vi "get_ID.vi"(4 "temps d'observation (ms)":u32=300, 6 "Log?":bool, 8 "errin":errorcluster, 10 "ChannelIn":T2, 11 "Identifier":u32 format="%x") -> (0 "errout":errorcluster, 1 "trouvé":bool, 2 "TimeStampOut":T1, 3 "Messout":T3)   [LabVIEW 2020]
uses:
  C/Program Files (x86)/National Instruments/LabVIEW 2020/user.lib/PCAN Basic/Controls/Channel.ctl
  FGV.ctl
  PCANBasic.dll
  C/Program Files (x86)/National Instruments/LabVIEW 2020/user.lib/PCAN Basic/PCANBasic.lvlib
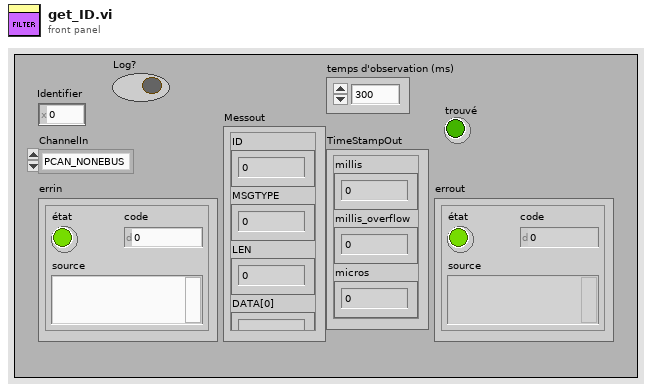
[diagram p1: front panel]
types:
  T1 = cluster{"millis":u32, "millis_overflow":u16, "micros":u16}
  T2 = typedef "PCANBasic.lvlib/Channel.ctl" = enum16{"PCAN_NONEBUS", "not used1", "not used2", "not used3", "not used4", "not used5", "not used6", "not used7", "not used8", "not used9", "not used10", "not used11", "not used12", "not used13", "not used14", "not used15", "not used16", "not used17", "not used18", "not used19", "not used20", "not used21", "not used22", "not used23", "not used24", "not used25", "not used26", "not used27", "not used28", "not used29", "not used30", "not used31", "not used32", "PCAN_ISABUS1", "PCAN_ISABUS2", "PCAN_ISABUS3", "PCAN_ISABUS4", "PCAN_ISABUS5", "PCAN_ISABUS6", "PCAN_ISABUS7", "PCAN_ISABUS8", "not used41", "not used42", "not used43", "not used44", "not used45", "not used46", "not used47", "not used48", "PCAN_DNGBUS1", "not used50", "not used51", "not used52", "not used53", "not used54", "not used55", "not used56", "not used57", "not used58", "not used59", "not used60", "not used61", "not used62", "not used63", "not used64", "PCAN_PCIBUS1", "PCAN_PCIBUS2", "PCAN_PCIBUS3", "PCAN_PCIBUS4", "PCAN_PCIBUS5", "PCAN_PCIBUS6", "PCAN_PCIBUS7", "PCAN_PCIBUS8", "not used73", "not used74", "not used75", "not used76", "not used77", "not used78", "not used79", "not used80", "PCAN_USBBUS1", "PCAN_USBBUS2", "PCAN_USBBUS3", "PCAN_USBBUS4", "PCAN_USBBUS5", "PCAN_USBBUS6", "PCAN_USBBUS7", "PCAN_USBBUS8", "Not used89", "Not used90", "Not used91", "Not used92", "Not used93", "Not used94", "Not used95", "Not used96", "PCAN_PCCBUS1", "PCAN_PCCBUS2"}
  T3 = cluster{"ID":u32, "MSGTYPE":u8, "LEN":u8, "DATA[0]":u8, "DATA[1]":u8, "DATA[2]":u8, "DATA[3]":u8, "DATA[4]":u8, "DATA[5]":u8, "DATA[6]":u8, "DATA[7]":u8}
  T4 = typedef "FGV.ctl" = enum16{"GET", "SET", "RAZ"}
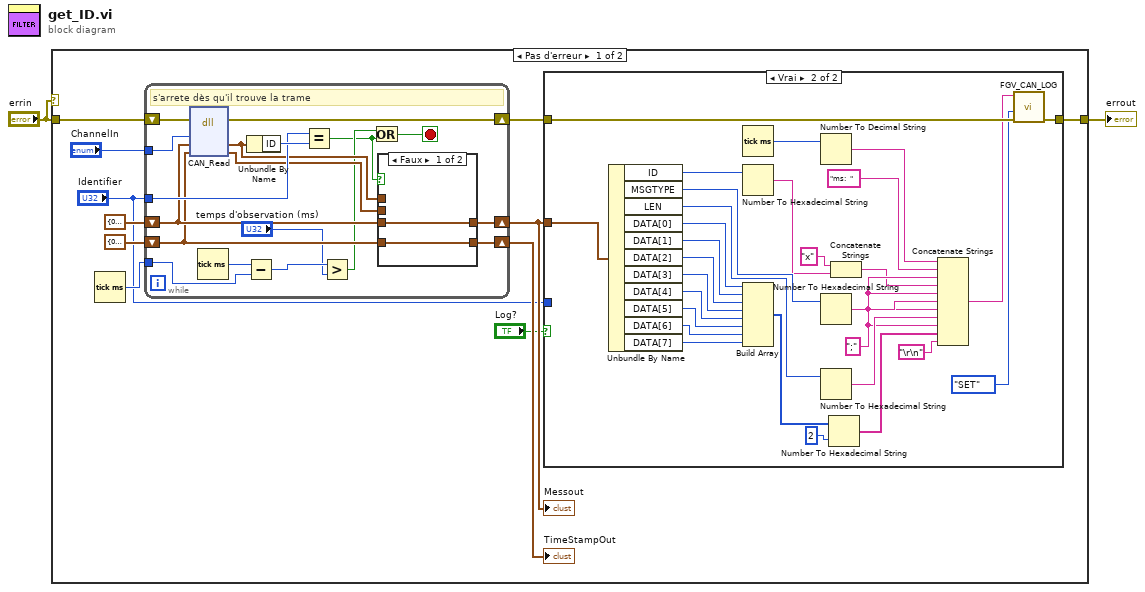
[diagram p0: block diagram]
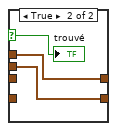
[diagram p3: hidden frame]
diagram:
  n1 = case shown="Pas d'erreur" "errin" {
    tunnel: "errin" -> [w13 w67]
    tunnel: [w6 w67] -> w2
    frame No Error {
      n2 = Tick Count (ms)() -> (millisecond timer value=w8:u32)
      n3 = while {
        tunnel: "ChannelIn" -> [w61]
        shift-right: [w59] -> w7
        shift-left: w13 -> [w60]
        tunnel: "Identifier" -> [w57]
        shift-right: [w56] -> w5
        shift-left: T3 {"ID"=0, "MSGTYPE"=0, "LEN"=0, "DATA[0]"=0, "DATA[1]"=0, "DATA[2]"=0, "DATA[3]"=0, "DATA[4]"=0, "DATA[5]"=0, "DATA[6]"=0, "DATA[7]"=0} ("MessageBuffer out") -> [w54]
        shift-right: [w55] -> w9
        shift-left: T1 {"millis"=0, "millis_overflow"=0, "micros"=0} ("TimestampBuffer out 2") -> [w53]
        tunnel: w8 -> [w50]
        stop <- w44 stop-if-true
        # "s'arrete dès qu'il trouve la trame"
        n4 = dll-call lib="PCANBasic.*" fn="CAN_Read"(error in=w60, "Channel"=w61, "MessageBuffer out"=w54, "TimestampBuffer out 2"=w53) -> (error out=w59:errorcluster, "MessageBuffer out"=w52:T3, "TimestampBuffer out 2"=w47:T1)  [unwired: 4 in, 1 out]
        n5 = Tick Count (ms)() -> (millisecond timer value=w51:u32)
        n6 = Subtract(x=w51, y=w50) -> (x-y=w49:u32)
        n7 = Unbundle By Name(w52) -> ("ID"=w58:u32)
        n8 = Equal?(x=w57, y=w58) -> (x = y?=w45:bool)
        n9 = Greater?(x=w49, y="temps d'observation (ms)") -> (0:w46:bool)
        n10 = Or(x=w46, y=w45) -> (x .or. y?=w44:bool)
        n11 = case shown="Faux" w45 {
          selector: w45 -> [_ w64]
          tunnel: w54 -> [w63 _]
          tunnel: [w63 w66] -> w56
          tunnel: [w62 w65] -> w55
          tunnel: w53 -> [w62 _]
          tunnel: w52 -> [_ w66]
          tunnel: w47 -> [_ w65]
          frame False {
          }
          frame True {
            "trouvé" <- w64
          }
        }
      }
      "Messout" <- w5
      "TimeStampOut" <- w9
      n12 = case shown="Vrai" "Log?" {
        tunnel: w7 -> [w14 w43]
        tunnel: [w14 w42] -> w6
        tunnel: w5 -> [_ w41]
        tunnel: "Identifier" -> [_ _]
        frame False {
        }
        frame True {
          w21 = ";" ("chaîne")
          n13 = Unbundle By Name(w41) -> ("ID"=w40:u32, "MSGTYPE"=w38:u8, "LEN"=w37:u8, "DATA[0]"=w34:u8, "DATA[1]"=w33:u8, "DATA[2]"=w32:u8, "DATA[3]"=w31:u8, "DATA[4]"=w30:u8, "DATA[5]"=w27:u8, "DATA[6]"=w28:u8, "DATA[7]"=w29:u8)
          n14 = Tick Count (ms)() -> (millisecond timer value=w39:u32)
          n15 = Number To Hexadecimal String(2:w40) -> (0:w16:string)  [unwired: 1 in]
          n16 = Build Array(w34, w33, w32, w31, w30, w27, w28, w29) -> (w25:u8[])
          n17 = Number To Decimal String(number=w39) -> (decimal integer string=w20:string)  [unwired: 1 in]
          n18 = Number To Hexadecimal String(2:w38) -> (0:w36:string)  [unwired: 1 in]
          n19 = Number To Hexadecimal String(2:w37) -> (0:w35:string)  [unwired: 1 in]
          n20 = Number To Hexadecimal String(1:i16 2 ("largeur (-)"), 2:w25) -> (0:w24:string[])
          n21 = Concatenate Strings("x" ("chaîne"), w16) -> (w15:string)
          n22 = Concatenate Strings(w20, "ms:  " ("chaîne"), w21, w15, w21, w36, w21, w35, w21, w24, "\r\n") -> (w23:string)
          n23 = call "FGV_CAN_LOG.vi"("errin"=w43, "CMD"=FGV."SET", "ChaineIn"=w23) -> ("errout"=w42:errorcluster)  [unwired: 7 in, 1 out]
        }
      }
    }
    frame Error {
    }
  }
  "errout" <- w2
